vi "etlWriteFuncGen.vi"(1 "lens":enum16{"0", "1"}(ring)) -> ()   [LabVIEW 2017]
uses:
  <vilib>/DAQmx/write.llb/DAQmx Write (Analog 1D DBL 1Chan NSamp).vi
  globalDevices.vi
  globalUtilities.vi
  <vilib>/DAQmx/miscellaneous.llb/DAQmx Fill In Error Info.vi
panel:
  out "success":bool
  out "Waveform Graph 3":dbl[](graph)
  out "nT":i32
  out "dt":dbl
  out "omega":dbl
  out "amplitude":dbl
  out "offset":dbl
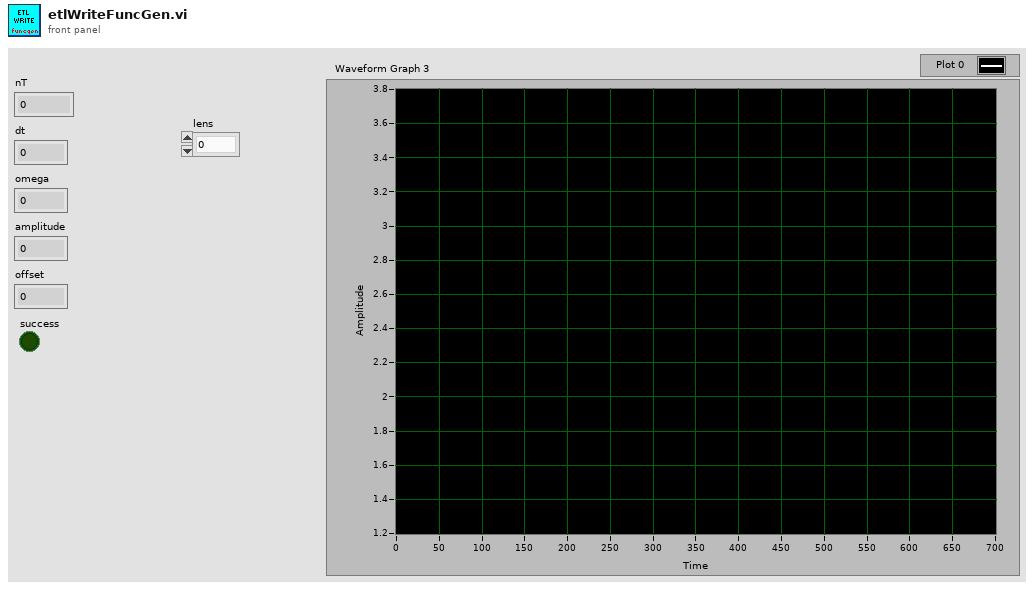
[diagram p1: front panel]
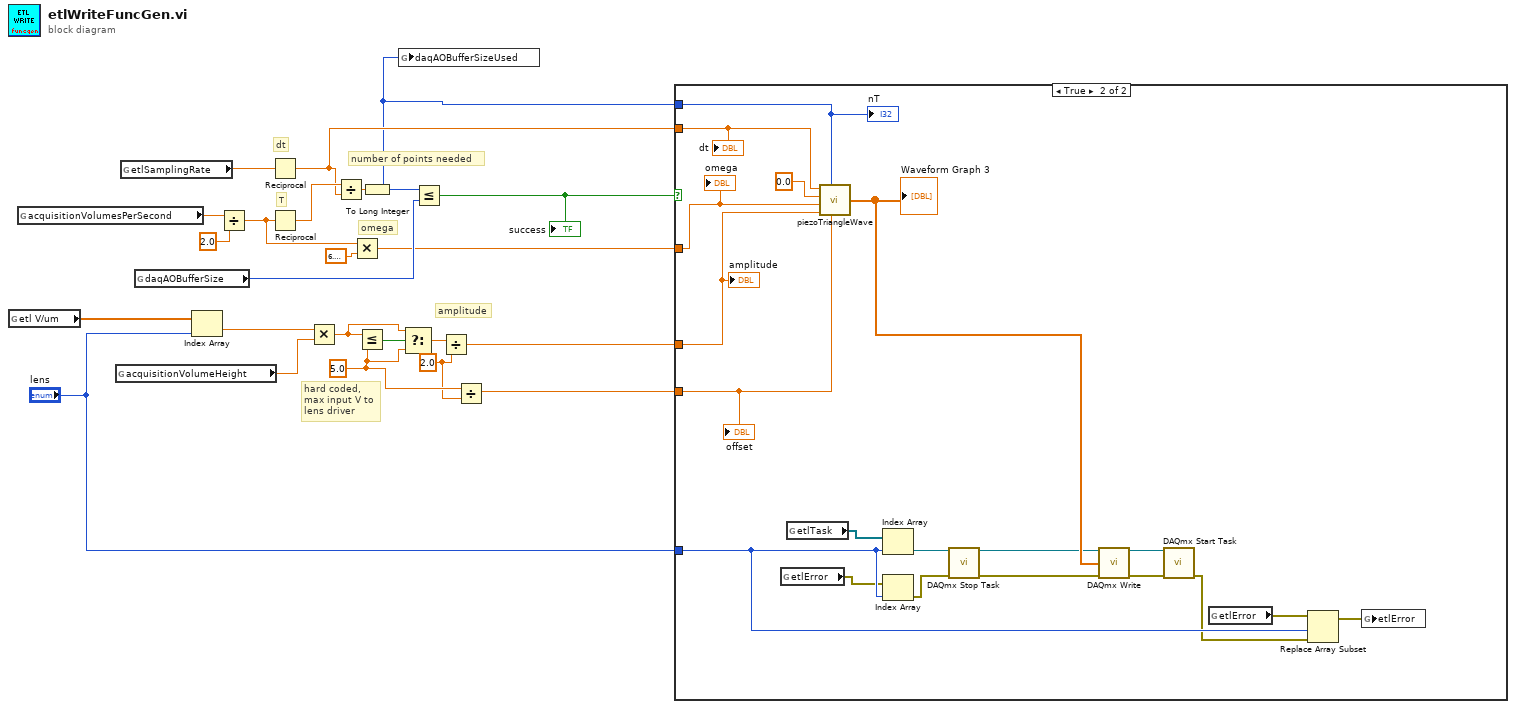
[diagram p0: block diagram]
diagram:
  w4 = 5.0 ("y")
  w3 = 2.0 ("y")
  # "hard coded,\nmax input V to\nlens driver"
  # "omega"
  # "amplitude"
  # "number of points needed"
  # "T"
  # "dt"
  n1 = global read "globalDevices.vi" "etl V/um"() -> (w6:dbl[])
  n2 = global read "globalUtilities.vi" "acquisitionVolumesPerSecond"() -> (w22:dbl)
  n3 = global read "globalUtilities.vi" "acquisitionVolumeHeight"() -> (w17:dbl)
  n4 = global read "globalDevices.vi" "etlSamplingRate"() -> (w23:dbl)
  n5 = global read "globalDevices.vi" "daqAOBufferSize"() -> (w19:i32)
  n6 = Index Array(array=w6, index="lens") -> (element=w5:dbl)
  n7 = Divide(x=w22, y=2.0) -> (x/y=w11:dbl)
  n8 = Reciprocal(x=w23) -> (1/x=w9:dbl)
  n9 = Reciprocal(x=w11) -> (1/x=w20:dbl)
  n10 = Multiply(x=w5, y=w17) -> (x*y=w15:dbl)
  n11 = Divide(x=w20, y=w9) -> (x/y=w8:dbl)
  n12 = Multiply(x=w11, y=6.283185307179586) -> (x*y=w10:dbl)
  n13 = Less Or Equal?(x=w15, y=w4) -> (x <= y?=w16:bool)
  n14 = To Long Integer(number=w8) -> (32bit integer=w7:i32)
  n15 = global write "globalDevices.vi" "daqAOBufferSizeUsed"(w7) -> ()
  n16 = Select(t=w15, s=w16, f=w4) -> (s? t:f=w14:dbl)
  n17 = Less Or Equal?(x=w7, y=w19) -> (x <= y?=w18:bool)
  "success" <- w18
  n18 = Divide(x=w14, y=w3) -> (x/y=w13:dbl)
  n19 = Divide(x=w4, y=w3) -> (x/y=w2:dbl)
  n20 = case shown="True" w18 {
    tunnel: w13 -> [_ w38]
    tunnel: w2 -> [_ w37]
    tunnel: w10 -> [_ w39]
    tunnel: w7 -> [_ w41]
    tunnel: w9 -> [_ w40]
    tunnel: "lens" -> [_ w36]
    frame False {
    }
    frame True {
      n21 = global read "globalDevices.vi" "etlError"() -> (w29:errorcluster[])
      n22 = global read "globalDevices.vi" "etlTask"() -> (w30:refnum<k21>[])
      n23 = call "piezoTriangleWave.vi"("offset"=w37, "nT"=w41, "amplitude"=w38, "omega"=w39, "t0"=0.0, "dt"=w40) -> ("x+y"=w35:dbl[])
      "Waveform Graph 3" <- w35
      n24 = Index Array(array=w30, index=w36) -> (element=w28:refnum<k21>)
      n25 = Index Array(array=w29, index=w36) -> (element=w27:errorcluster)
      n26 = call <vilib>:"DAQmx Stop Task.vi"("task/channels in"=w28, "error in"=w27) -> ("task out"=w31:refnum<k21>, "error out"=w32:errorcluster)  [unwired: 12 in]
      n27 = call-poly <vilib>:"DAQmx Write.vi"("task/channels in"=w31, "data"=w35, "error in"=w32) -> ("task out"=w33:refnum<k21>, "error out"=w34:errorcluster)  [unwired: 10 in, 1 out]
      n28 = call <vilib>:"DAQmx Start Task.vi"("task/channels in"=w33, "error in"=w34) -> ("error out"=w25:errorcluster)  [unwired: 12 in, 1 out]
      n29 = global read "globalDevices.vi" "etlError"() -> (w26:errorcluster[])
      n30 = Replace Array Subset(array=w26, new element=w25, index=w36) -> (w24:errorcluster[])
      n31 = global write "globalDevices.vi" "etlError"(w24) -> ()
      "nT" <- w41
      "dt" <- w40
      "omega" <- w39
      "amplitude" <- w38
      "offset" <- w37
    }
  }
